vi "Configure Auto Level Control.vi"(8 "error in (no error)":errorcluster, 10 "Auto Level Control (F:Disable)":bool, 11 "VISA resource name":refnum<visa-resource-name>) -> (0 "error out":errorcluster, 3 "VISA resource name out":refnum<visa-resource-name>)   [LabVIEW 2017, in "Agilent E4980.lvlib"]
doc: "The automatic level control (ALC) function adjusts the signal across the DUT to the same level as the voltage or current level setting. Using this feature, you can maintain a constant level (voltage or current) of measurement signals applied to the DUT.\n\nThe automatic level control feature uses a monitorable feedback circuit, and iterates a feedback loop that consists of level measurement and level change. The loop works two to nine times every measurement cycle. (The time required for level adjustment depends on how many times the feedback loop is iterated (the value \"n\"), and in turn, the value \"n\" depends on the characteristics of the DUT)"
uses:
  Agilent E4980.lvlib
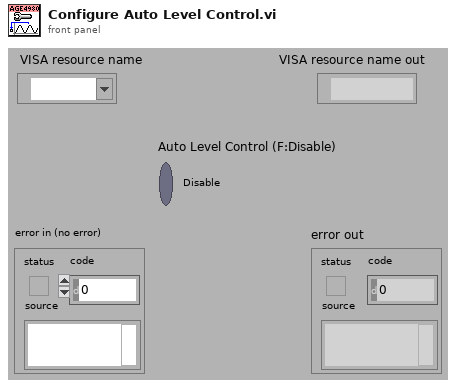
[diagram p1: front panel]
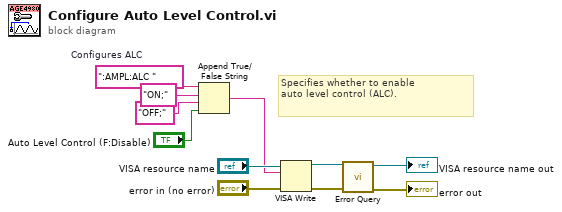
[diagram p0: block diagram]
diagram:
  w11 = ":AMPL:ALC "  # Configures ALC
  # "Specifies whether to enable\nauto level control (ALC)."
  n1 = Append True/False String(1:"Auto Level Control (F:Disable)", 2:"OFF;" ("false string"), 3:"ON;" ("true string"), 4:w11) -> (0:w6:string)
  n2 = VISA Write(VISA resource name="VISA resource name", write buffer=w6, error in (no error)="error in (no error)") -> (VISA resource name out=w5:refnum<visa-resource-name>, error out=w4:errorcluster)  [unwired: 1 out]
  n3 = call "Error Query.vi"("error in (no error)"=w4, "VISA resource name"=w5) -> ("error out"=→"error out":errorcluster, "VISA resource name out"=→"VISA resource name out":refnum<visa-resource-name>)  [unwired: 6 in, 2 out]
